vi "Select DaisyChain device.vi"(0 "System no.":i32=1 min=1 max=4 step=1, 1 "DLL Interface":T1=5 items=["RS232", "GPIB", "Board", "TCP-IP", "USB", "RS232_DC", "USB_DC", "TCPIP_DC"], 2 "Controller name":string, 3 "Timeout":i32=5000, 4 "Register DC":bool, 5 "error in":errorcluster, 6 "RS232 Portnumber":i32(ring) items=["COM1", "COM2", "COM3", "COM4", "COM5", "COM6", "COM7", "COM8", "COM9", "COM10", "COM11", "COM12", "COM13", "COM14", "COM15", "COM16", "COM17", "COM18", "COM19", "COM20", "COM21", "COM22", "COM23", "COM24", "COM25", "COM26", "COM27", "COM28", "COM29", "COM30"], 7 "RS232 Baud rate":i32=57600, 8 "Parameter":string) -> (14 "Selected DaisyChain controller":string, 15 "DeviceID out":i32, 19 "error out":errorcluster)   [LabVIEW 2026]
doc: "Performs a broadcast, returns names of all controllers matching Controller name and lets the user select the appropriate controller from a ring control. VI will also stop if Cancel is TRUE.\n\nC-867: Controller name = \"C-867\", DLL Interface = RS232_DC\nC-885: Controller name = \"C-885\", DLL Interface = USB_DC or TCPIP_DC\nE-709: Controller name = \"E-709\", DLL Interface = RS232_DC. Only supported if E-709 is used inside C-867K012/K013.\nE-755: Controller name = \"E-755\", DLL Interface = RS232_DC\nE-861: Controller name = \"E-861\", DLL Interface = RS232_DC or USB_DC\nE-871: Controller name = \"E-871\", DLL Interface = RS232_DC or USB_DC\nMercury_GCS: Controller name = \"Mercury_GCS\", DLL Interface = RS232_DC or USB_DC"
uses:
  Available DLL interfaces.ctl
  Available interfaces.ctl
  Available DLLs.ctl
  Global1.vi
  Global DaisyChain.vi
panel:
  in  "abort":bool
  in  "ok":bool
  in  "Please select DaisyChain controller":u16(ring) items=["DeviceID 1: (c)2013 Physik Instrumente (PI) GmbH & Co. KG, E-871.1A1, 0, 01.009 ", "DeviceID 2: <device 2 not connected> ", "DeviceID 3: <device 3 not connected> ", "DeviceID 4: <device 4 not connected> ", "DeviceID 5: <device 5 not connected> ", "DeviceID 6: <device 6 not connected> ", "DeviceID 7: <device 7 not connected> ", "DeviceID 8: <device 8 not connected> ", "DeviceID 9: (c)2013 Physik Instrumente (PI) GmbH & Co. KG, E-871.1A1, 0, 01.009 ", "DeviceID 10: <device 10 not connected> ", "DeviceID 11: <device 11 not connected> ", "DeviceID 12: <device 12 not connected> ", "DeviceID 13: <device 13 not connected> ", "DeviceID 14: <device 14 not connected> ", "DeviceID 15: <device 15 not connected> ", "DeviceID 16: <device 16 not connected> ", "DeviceID 17: <device 17 not connected>"]
  out "Please wait":string="Broadcast is running, please wait..."
  # "Scan parameters and controller name to search for:"
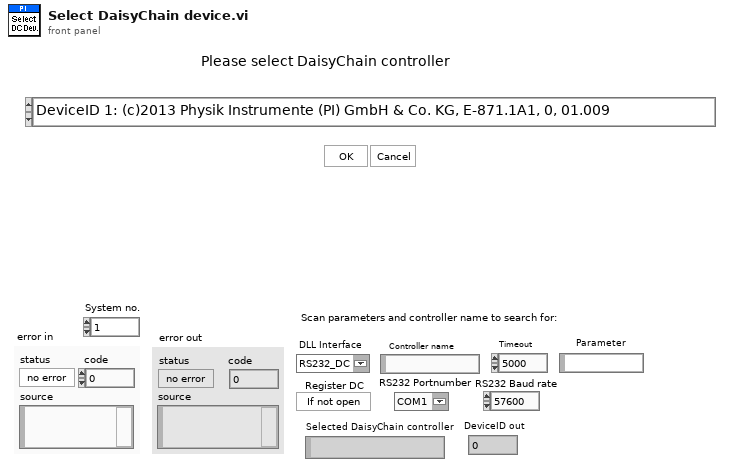
[diagram p1: front panel]
types:
  T1 = typedef "Available DLL interfaces.ctl" = u16
  T2 = enum16{"C844_IsDLLAvailable", "C844_ConnectRS232", "C844_ConnectNIgpib", "C844_IsConnected", "C844_CloseConnection", "C844_GcsCommandset", "C844_GetError", "C844_GcsGetAnswerSize", "C844_GcsGetAnswer", "C843_IsDLLAvailable", "C843_Connect", "C843_IsConnected", "C843_CloseConnection", "C843_GcsCommandset", "C843_GetError", "C843_GcsGetAnswerSize", "C843_GcsGetAnswer", "E710_IsDLLAvailable", "E710_ConnectRS232", "E710_ConnectNIgpib", "E710_IsConnected", "E710_CloseConnection", "E710_GcsCommandset", "E710_GetError", "E710_GcsGetAnswerSize", "E710_GcsGetAnswer", "C843_PM_IsDLLAvailable", "C843_PM_Connect", "C843_PM_IsConnected", "C843_PM_CloseConnection", "C843_PM_GcsCommandset", "C843_PM_GetError", "C843_PM_GcsGetAnswerSize", "C843_PM_GcsGetAnswer", "C843_PM_GetCurrentBoardID", "C843_GetCurrentBoardID", "C865_IsDLLAvailable", "C865_ConnectRS232", "C865_IsConnected", "C865_CloseConnection", "C865_GcsCommandset", "C865_GetError", "C865_GcsGetAnswerSize", "C865_GcsGetAnswer", "C865_GetCurrentInterfaceID", "E761_ConnectPciBoard", "DefineSystem", "CloseConnection", "IsConnected", "ConnectRS232", "ConnectNIgpib", "ConnectPciBoard", "ConnectTCPIP", "GetError", "GcsCommandset", "GCSGetAnswerSize", "GcsGetAnswer"}
  T3 = enum16{"C844_IsDLLAvailable", "C844_ConnectRS232", "C844_ConnectNIgpib", "C844_IsConnected", "C844_CloseConnection", "C844_GcsCommandset", "C844_GetError", "C844_GcsGetAnswerSize", "C844_GcsGetAnswer", "C843_IsDLLAvailable", "C843_Connect", "C843_IsConnected", "C843_CloseConnection", "C843_GcsCommandset", "C843_GetError", "C843_GcsGetAnswerSize", "C843_GcsGetAnswer", "E710_IsDLLAvailable", "E710_ConnectRS232", "E710_ConnectNIgpib", "E710_IsConnected", "E710_CloseConnection", "E710_GcsCommandset", "E710_GetError", "E710_GcsGetAnswerSize", "E710_GcsGetAnswer", "C843_PM_IsDLLAvailable", "C843_PM_Connect", "C843_PM_IsConnected", "C843_PM_CloseConnection", "C843_PM_GcsCommandset", "C843_PM_GetError", "C843_PM_GcsGetAnswerSize", "C843_PM_GcsGetAnswer", "C843_PM_GetCurrentBoardID", "C843_GetCurrentBoardID", "C865_IsDLLAvailable", "C865_ConnectRS232", "C865_IsConnected", "C865_CloseConnection", "C865_GcsCommandset", "C865_GetError", "C865_GcsGetAnswerSize", "C865_GcsGetAnswer", "C865_GetCurrentInterfaceID", "E761_ConnectPciBoard", "DefineSystem", "CloseConnection", "IsConnected", "ConnectRS232", "ConnectNIgpib", "ConnectPciBoard", "ConnectTCPIP", "GetError", "GcsCommandset", "GCSGetAnswerSize", "GcsGetAnswer", "CloseDaisyChain", "OpenRS232DaisyChain", "ConnectDaisyChainDevice", "ConnectUSB", "ListUSB", "OpenUSBDaisyChain", "OpenTCPIPDaisyChain"}
  T4 = typedef "Available interfaces.ctl" = u16
  T5 = typedef "Available DLLs.ctl" = u16
  T6 = cluster{"DLL for Device":T5, "DLL Interface":T1, "Parameter":string}[]
  T7 = cluster{"RS232 Portnumber":i32, "Timeout":i32, "RS232 Baud rate":u32, "Interface":T4, "GPIB Bus":i32, "GPIB Address":i32, "GPIB Mode":i32}[]
  T8 = cluster{"input XON/XOFF":bool, "input HW Handshake":bool, "input alt HW HShk":bool, "output XON/XOFF":bool, "output HW Handshake":bool, "output alt HW HShk":bool, "XOFF byte ":u8, "XON byte":u8, "parity error byte":u16}[]
  T9 = cluster{"RS232 Portnumber":i32, "Timeout":i32, "RS232 Baud rate":u32, "Interface":T4, "GPIB Bus":i32, "GPIB Address":i32, "GPIB Mode":i32}
  T10 = cluster{"DLL for Device":T5, "DLL Interface":T1, "Parameter":string}
  T11 = cluster{"input XON/XOFF":bool, "input HW Handshake":bool, "input alt HW HShk":bool, "output XON/XOFF":bool, "output HW Handshake":bool, "output alt HW HShk":bool, "XOFF byte ":u8, "XON byte":u8, "parity error byte":u16}
  T12 = cluster{"No. of devices":i32, "Port ID":i32, "Devices":string[], "Description":string}[]
  T13 = cluster{"No. of devices":i32, "Port ID":i32, "Devices":string[], "Description":string}
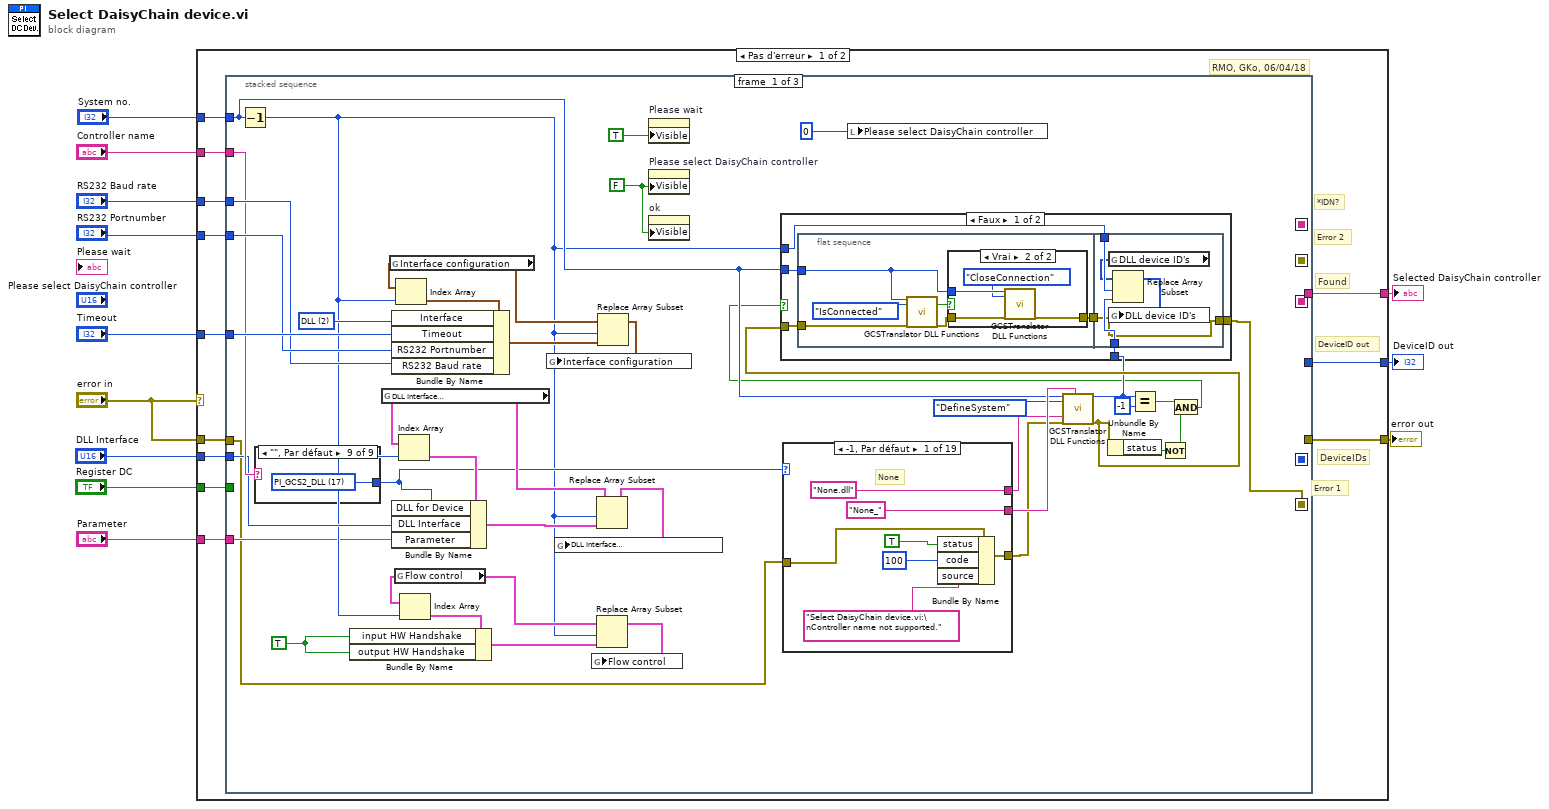
[diagram p0: block diagram]
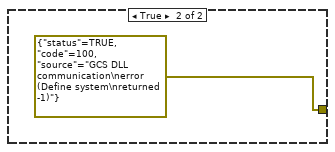
[diagram p3: hidden frame]
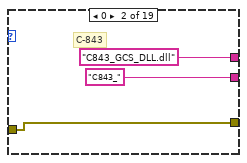
[diagram p4: hidden frame]
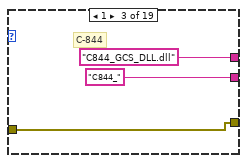
[diagram p5: hidden frame]
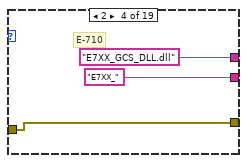
[diagram p6: hidden frame]
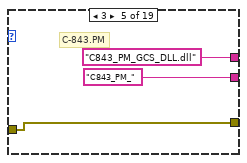
[diagram p7: hidden frame]
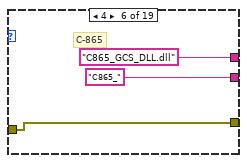
[diagram p8: hidden frame]
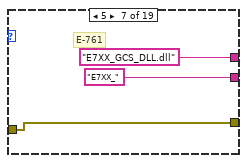
[diagram p9: hidden frame]
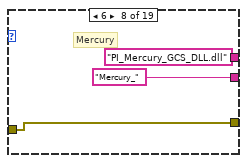
[diagram p10: hidden frame]
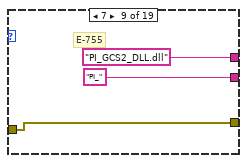
[diagram p11: hidden frame]
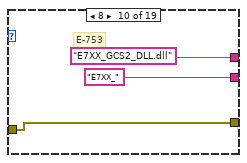
[diagram p12: hidden frame]
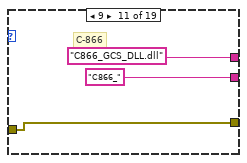
[diagram p13: hidden frame]
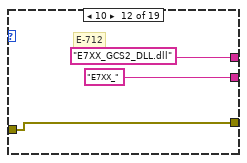
[diagram p14: hidden frame]
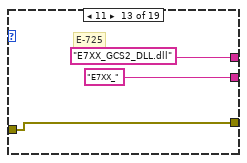
[diagram p15: hidden frame]
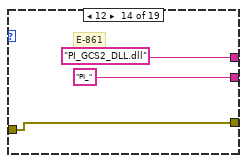
[diagram p16: hidden frame]
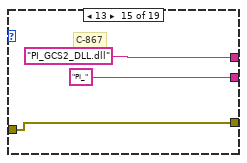
[diagram p17: hidden frame]
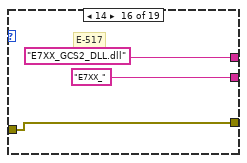
[diagram p18: hidden frame]
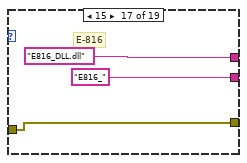
[diagram p19: hidden frame]
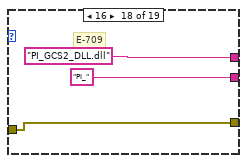
[diagram p20: hidden frame]
diagram:
  n1 = case shown="Pas d'erreur" "error in" {
    tunnel: [w21 w360] -> w12
    tunnel: "error in" -> [w22 w360]
    tunnel: "RS232 Baud rate" -> [w24 _]
    tunnel: "Controller name" -> [w23 _]
    tunnel: [w19 "" ("Host address/name")] -> w8
    tunnel: "RS232 Portnumber" -> [w20 _]
    tunnel: [w18 0] -> w7
    tunnel: "Register DC" -> [w17 _]
    tunnel: "System no." -> [w16 _]
    tunnel: "Timeout" -> [w15 _]
    tunnel: "DLL Interface" -> [w14 _]
    tunnel: "Parameter" -> [w13 _]
    frame No Error {
      # "DeviceIDs"
      # "Error 1"
      # "DeviceID out"
      # "Error 2"
      # "Found"
      # "*IDN?"
      # "RMO, GKo, 06/04/18"
      n2 = stacked-sequence {
        seq-local: [_ w163 _] -> [_ _ w304]
        seq-local: [_ w165 _] -> [_ _ w307]
        seq-local: [_ w161 _] -> [_ _ w302]
        seq-local: [w29 _ _] -> [_ w157 _]
        seq-local: [_ w159 _] -> [_ _ w301]
        tunnel: w24 -> [w53 _ _]
        tunnel: w23 -> [w51 w164 _]
        tunnel: w22 -> [w26 _ _]
        tunnel: [_ _ w303] -> w21
        tunnel: [_ _ w306] -> w19
        tunnel: w20 -> [w54 _ _]
        tunnel: [_ _ w305] -> w18
        tunnel: w17 -> [_ w162 _]
        tunnel: w16 -> [w33 w160 _]
        tunnel: w15 -> [w58 _ _]
        tunnel: w14 -> [w50 w158 _]
        tunnel: w13 -> [w27 _ _]
        frame #0 {
          w43 = FALSE ("Visible")
          w62 = T4 2 items=["RS232", "GPIB", "DLL", "TCP-IP"] ("Interface")
          w60 = TRUE ("Bundle Element")
          n3 = Decrement(x=w33) -> (x-1=w31:i32)
          n4 = case shown="\"\", Par défaut" w51 {
            tunnel: [-1 w149 w150 w151 w152 w153 w154 w155 w156] -> w37
            frame "None" {
            }
            frame "E-755" {
              w149 = T5 7 items=["C-843", "C-844", "E-710", "C-843.PM", "C-865", "E-761", "Mercury", "E-755", "E-753", "C-866", "E-712", "E-725", "E-861", "C-867", "E-517", "E-816", "E-709", "PI_GCS2_DLL", "HydraPollux"] ("DLL for Device")
            }
            frame "E-861" {
              w150 = T5 12 items=["C-843", "C-844", "E-710", "C-843.PM", "C-865", "E-761", "Mercury", "E-755", "E-753", "C-866", "E-712", "E-725", "E-861", "C-867", "E-517", "E-816", "E-709", "PI_GCS2_DLL", "HydraPollux"] ("DLL for Device")
            }
            frame "E-709" {
              w151 = T5 17 items=["C-843", "C-844", "E-710", "C-843.PM", "C-865", "E-761", "Mercury", "E-755", "E-753", "C-866", "E-712", "E-725", "E-861", "C-867", "E-517", "E-816", "E-709", "PI_GCS2_DLL", "HydraPollux"] ("DLL for Device")
            }
            frame "C-867" {
              w152 = T5 13 items=["C-843", "C-844", "E-710", "C-843.PM", "C-865", "E-761", "Mercury", "E-755", "E-753", "C-866", "E-712", "E-725", "E-861", "C-867", "E-517", "E-816", "E-709", "PI_GCS2_DLL", "HydraPollux"] ("DLL for Device")
            }
            frame "Mercury_GCS" {
              w153 = T5 17 items=["C-843", "C-844", "E-710", "C-843.PM", "C-865", "E-761", "Mercury", "E-755", "E-753", "C-866", "E-712", "E-725", "E-861", "C-867", "E-517", "E-816", "E-709", "PI_GCS2_DLL", "HydraPollux"] ("DLL for Device")
            }
            frame "E-871" {
              w154 = T5 17 items=["C-843", "C-844", "E-710", "C-843.PM", "C-865", "E-761", "Mercury", "E-755", "E-753", "C-866", "E-712", "E-725", "E-861", "C-867", "E-517", "E-816", "E-709", "PI_GCS2_DLL", "HydraPollux"] ("DLL for Device")
            }
            frame "C-885" {
              w155 = T5 17 items=["C-843", "C-844", "E-710", "C-843.PM", "C-865", "E-761", "Mercury", "E-755", "E-753", "C-866", "E-712", "E-725", "E-861", "C-867", "E-517", "E-816", "E-709", "PI_GCS2_DLL", "HydraPollux"] ("DLL for Device")
            }
            frame "", Default {
              w156 = T5 17 items=["C-843", "C-844", "E-710", "C-843.PM", "C-865", "E-761", "Mercury", "E-755", "E-753", "C-866", "E-712", "E-725", "E-861", "C-867", "E-517", "E-816", "E-709", "PI_GCS2_DLL", "HydraPollux"] ("DLL for Device")
            }
          }
          n5 = global read "Global1.vi" "DLL Interface\nConfiguration"() -> (w46:T6)
          n6 = global read "Global1.vi" "Interface configuration"() -> (w47:T7)
          n7 = global read "Global1.vi" "Flow control"() -> (w45:T8)
          n8 = Index Array(array=w47, index=w31) -> (element=w63:T9)
          n9 = Bundle By Name(cluster=w63, "Interface"=w62, "Timeout"=w58, "RS232 Portnumber"=w54, "RS232 Baud rate"=w53) -> (w52:T9)
          n10 = Index Array(array=w46, index=w31) -> (element=w59:T10)
          n11 = Bundle By Name(cluster=w59, "DLL for Device"=w37, "DLL Interface"=w50, "Parameter"=w27) -> (w49:T10)
          n12 = Index Array(array=w45, index=w31) -> (element=w61:T11)
          n13 = Bundle By Name(cluster=w61, "input HW Handshake"=w60, "output HW Handshake"=w60) -> (w48:T11)
          n14 = Replace Array Subset(array=w46, new element=w49, index=w31) -> (w56:T6)
          n15 = global write "Global1.vi" "DLL Interface\nConfiguration"(w56) -> ()
          n16 = Replace Array Subset(array=w45, new element=w48, index=w31) -> (w57:T8)
          n17 = global write "Global1.vi" "Flow control"(w57) -> ()
          n18 = Replace Array Subset(array=w47, new element=w52, index=w31) -> (w55:T7)
          n19 = global write "Global1.vi" "Interface configuration"(w55) -> ()
          n20 = property on="Please wait" class="Ch"("Visible"=TRUE) -> ()  [unwired: 2 in, 2 out]
          n21 = property on="Please select DaisyChain controller" class="MDér (strict)"("Visible"=w43) -> ()  [unwired: 2 in, 2 out]
          n22 = property on="ok" class="Bool"("Visible"=w43) -> ()  [unwired: 2 in, 2 out]
          n23 = case shown="-1, Par défaut" w37 {
            tunnel: ["None.dll" "C843_GCS_DLL.dll" "C844_GCS_DLL.dll" "E7XX_GCS_DLL.dll" "C843_PM_GCS_DLL.dll" "C865_GCS_DLL.dll" "E7XX_GCS_DLL.dll" "PI_Mercury_GCS_DLL.dll" "PI_GCS2_DLL.dll" "E7XX_GCS2_DLL.dll" "C866_GCS_DLL.dll" "E7XX_GCS2_DLL.dll" "E7XX_GCS2_DLL.dll" "PI_GCS2_DLL.dll" "PI_GCS2_DLL.dll" "E7XX_GCS2_DLL.dll" "E816_DLL.dll" "PI_GCS2_DLL.dll" "PI_GCS2_DLL.dll"] -> w40
            tunnel: ["None_" "C843_" "C844_" "E7XX_" "C843_PM_" "C865_" "E7XX_" "Mercury_" "PI_" "E7XX_" "C866_" "E7XX_" "E7XX_" "PI_" "PI_" "E7XX_" "E816_" "PI_" "PI_"] -> w41
            tunnel: w26 -> [w87 w94 w97 w100 w103 w106 w109 w112 w115 w118 w121 w124 w127 w130 w133 w136 w139 w142 w145]
            tunnel: [w91 w94 w97 w100 w103 w106 w109 w112 w115 w118 w121 w124 w127 w130 w133 w136 w139 w142 w145] -> w25
            frame -1, Default {
              # "None"
              n24 = Bundle By Name(cluster=w87, "status"=TRUE, "code"=100, "source"="Select DaisyChain device.vi:\nController name not supported.") -> (w91:errorcluster)
            }
            frame 0 {
              # "C-843"
            }
            frame 1 {
              # "C-844"
            }
            frame 2 {
              # "E-710"
            }
            frame 3 {
              # "C-843.PM"
            }
            frame 4 {
              # "C-865"
            }
            frame 5 {
              # "E-761"
            }
            frame 6 {
              # "Mercury"
            }
            frame 7 {
              # "E-755"
            }
            frame 8 {
              # "E-753"
            }
            frame 9 {
              # "C-866"
            }
            frame 10 {
              # "E-712"
            }
            frame 11 {
              # "E-725"
            }
            frame 12 {
              # "E-861"
            }
            frame 13 {
              # "C-867"
            }
            frame 14 {
              # "E-517"
            }
            frame 15 {
              # "E-816"
            }
            frame 16 {
              # "E-709"
            }
            frame 17 {
              # "PI_GCS2_DLL"
            }
          }
          n25 = local write "Please select DaisyChain controller"(0) -> ()
          n26 = call "GCSTranslator DLL Functions.vi"("System no."=w33, "Function"=T2."DefineSystem", "String input"=w40, "error in"=w25, "String input 2"=w41) -> ("DLL I32 Return value"=w30:i32, "error out"=w32:errorcluster)  [unwired: 2 in, 11 out]
          n27 = Unbundle By Name(w32) -> ("status"=w35:bool)
          n28 = Equal?(x=w30, y=-1) -> (x = y?=w36:bool)
          n29 = Not(x=w35) -> (.not. x?=w34:bool)
          n30 = And(x=w36, y=w34) -> (x .and. y?=w28:bool)
          n31 = case shown="Faux" w28 {
            tunnel: w33 -> [w64 _]
            tunnel: w32 -> [w67 _]
            tunnel: w31 -> [w69 _]
            tunnel: w30 -> [w68 _]
            tunnel: [w65 errorcluster {"status"=TRUE, "code"=100, "source"="GCS DLL communication\nerror (Define system\nreturned -1)"} ("error out")] -> w29
            frame False {
              n32 = flat-sequence {
                tunnel: w67 -> [w72]
                tunnel: [w71] -> w66
                tunnel: w64 -> [w70]
                tunnel: w69 -> [w85]
                tunnel: w68 -> [w82]
                tunnel: w66 -> [w81]
                tunnel: [w81] -> w65
                frame #0 {
                  n33 = call "GCSTranslator DLL Functions.vi"("System no."=w70, "Function"=T2."IsConnected", "error in"=w72) -> ("Boolean output"=w75:bool, "error out"=w74:errorcluster)  [unwired: 4 in, 11 out]
                  n34 = case shown="Vrai" w75 {
                    tunnel: w70 -> [_ w80]
                    tunnel: w74 -> [w76 w79]
                    tunnel: [w76 w78] -> w71
                    frame False {
                    }
                    frame True {
                      n35 = call "GCSTranslator DLL Functions.vi"("System no."=w80, "Function"=T2."CloseConnection", "error in"=w79) -> ("error out"=w78:errorcluster)  [unwired: 4 in, 12 out]
                    }
                  }
                }
                frame #1 {
                  n36 = global read "Global1.vi" "DLL device ID's"() -> (w83:i32[])
                  n37 = Replace Array Subset(array=w83, new element=w82, index=w85) -> (w84:i32[])
                  n38 = global write "Global1.vi" "DLL device ID's"(w84) -> ()
                }
              }
            }
            frame True {
            }
          }
        }
        frame #1 {
          n39 = case shown="Pas d'erreur" w157 {
            tunnel: [w181 string[] []] -> w165
            tunnel: w164 -> [w167 _]
            tunnel: [w180 w300] -> w163
            tunnel: w162 -> [w179 _]
            tunnel: [w178 string[] []] -> w161
            tunnel: w160 -> [w173 _]
            tunnel: [w172 i32[] []] -> w159
            tunnel: w158 -> [w171 _]
            tunnel: w157 -> [w168 w300]
            frame No Error {
              n40 = Decrement(x=w173) -> (x-1=w177:i32)
              n41 = case shown="Vrai" w179 {
                tunnel: w168 -> [w256 w288]
                tunnel: [w252 w281] -> w170
                tunnel: w173 -> [w254 w286]
                tunnel: [w251 w283] -> w175
                tunnel: w177 -> [w250 _]
                tunnel: [w249 w284] -> w176
                tunnel: w171 -> [w248 w282]
                frame False {
                  n42 = call "Is DaisyChain open.vi"("System no."=w254, "error in"=w256) -> ("DC open?"=w255:bool, "error out"=w253:errorcluster)  [unwired: 16 out]
                  n43 = case shown="Faux" w255 {
                    tunnel: w254 -> [_ w270]
                    tunnel: w253 -> [w262 w269]
                    tunnel: [w262 w268] -> w252
                    tunnel: [w259 w267] -> w251
                    tunnel: w250 -> [w258 _]
                    tunnel: [w257 w265] -> w249
                    tunnel: w248 -> [_ w263]
                    frame True {
                      n44 = global read "Global DaisyChain.vi" "DaisyChain configuration"() -> (w260:T12)
                      n45 = Index Array(array=w260, index=w258) -> (element=w261:T13)
                      n46 = Unbundle By Name(w261) -> ("Port ID"=w259:i32, "Devices"=w257:string[])
                    }
                    frame False {
                      n47 = case shown="7" w263 {
                        tunnel: [T3."OpenRS232DaisyChain" ("Function") T3."OpenRS232DaisyChain" ("Function") T3."OpenRS232DaisyChain" ("Function") T3."OpenRS232DaisyChain" ("Function") T3."OpenRS232DaisyChain" ("Function") T3."OpenRS232DaisyChain" ("Function") T3."OpenUSBDaisyChain" ("Function") T3."OpenTCPIPDaisyChain" ("Function")] -> w264
                        frame 0, Default {
                        }
                        frame 1 {
                        }
                        frame 2 {
                        }
                        frame 3 {
                        }
                        frame 4 {
                        }
                        frame 5 {
                        }
                        frame 6 {
                        }
                        frame 7 {
                        }
                      }
                      n48 = call "GCSTranslator DLL Functions.vi"("System no."=w270, "Function"=w264, "error in"=w269) -> ("DLL I32 Return value"=w267:i32, "String output"=w266:string, "error out"=w268:errorcluster)  [unwired: 4 in, 10 out]
                      n49 = call "Get lines from string.vi"("Input string"=w266) -> ("Strings"=w265:string[])  [unwired: 2 in, 16 out]
                    }
                  }
                }
                frame True {
                  n50 = case shown="7" w282 {
                    tunnel: [T3."OpenRS232DaisyChain" ("Function") T3."OpenRS232DaisyChain" ("Function") T3."OpenRS232DaisyChain" ("Function") T3."OpenRS232DaisyChain" ("Function") T3."OpenRS232DaisyChain" ("Function") T3."OpenRS232DaisyChain" ("Function") T3."OpenUSBDaisyChain" ("Function") T3."OpenTCPIPDaisyChain" ("Function")] -> w280
                    frame 0, Default {
                    }
                    frame 1 {
                    }
                    frame 2 {
                    }
                    frame 3 {
                    }
                    frame 4 {
                    }
                    frame 5 {
                    }
                    frame 6 {
                    }
                    frame 7 {
                    }
                  }
                  n51 = call "GCSTranslator DLL Functions.vi"("System no."=w286, "Function"=T3."CloseDaisyChain", "error in"=w288) -> ("error out"=w287:errorcluster)  [unwired: 4 in, 12 out]
                  n52 = call "GCSTranslator DLL Functions.vi"("System no."=w286, "Function"=w280, "error in"=w287) -> ("DLL I32 Return value"=w283:i32, "String output"=w285:string, "error out"=w281:errorcluster)  [unwired: 4 in, 10 out]
                  n53 = call "Get lines from string.vi"("Input string"=w285) -> ("Strings"=w284:string[])  [unwired: 2 in, 16 out]
                }
              }
              n54 = case shown="\"Mercury_GCS\"" w167 {
                tunnel: [w183 string[] ["C-663", "C-863"]] -> w166
                tunnel: w167 -> [w182 _]
                frame Default {
                  n55 = Build Array(w182) -> (w183:string[])
                }
                frame "Mercury_GCS" {
                }
              }
              n56 = Not Equal?(x=w175, y=-1) -> (x != y?=w169:bool)
              n57 = case shown="Vrai" w169 {
                tunnel: [string[] [] w207] -> w181
                tunnel: w166 -> [_ w202]
                tunnel: [w187 w201] -> w180
                tunnel: [string[] [] w200] -> w178
                tunnel: w170 -> [w192 w199]
                tunnel: w176 -> [_ w198]
                tunnel: w173 -> [w191 _]
                tunnel: [i32[] [] w193] -> w172
                frame False {
                  # "Error!"
                  n58 = call "GCSTranslator DLL Functions.vi"("System no."=w191, "Function"=T3."GetError", "error in"=w192) -> ("error out"=w188:errorcluster)  [unwired: 4 in, 12 out]
                  n59 = call "GCSTranslateError.vi"("error in"=w188) -> ("error out"=w187:errorcluster)  [unwired: 18 out]
                }
                frame True {
                  n60 = for {
                    tunnel: w202 -> [w214] mode=indexing
                    tunnel: w198 -> [w212]
                    shift-right: [w213] -> w200
                    shift-left: string[] [] -> [w215]
                    shift-right: [w210] -> w194
                    shift-left: i32[] [] -> [w211]
                    n61 = for {
                      tunnel: w212 -> [w223] mode=indexing
                      shift-right: [w222] -> w213
                      shift-left: w215 -> [w221]
                      tunnel: w214 -> [w220]
                      shift-right: [w219] -> w210
                      shift-left: w211 -> [w218]
                      i -> [w216]
                      n62 = Match Pattern(string=w223, regular expression=w220) -> (offset past match=w217:i32)  [unwired: 4 out]
                      n63 = Not Equal?(x=w217, y=-1) -> (x != y?=w224:bool)
                      n64 = case shown="Vrai" w224 {
                        tunnel: w223 -> [_ w232]
                        tunnel: [w227 w233] -> w222
                        tunnel: w221 -> [w227 w231]
                        tunnel: [w226 w230] -> w219
                        tunnel: w218 -> [w226 w229]
                        tunnel: w216 -> [_ w228]
                        frame False {
                        }
                        frame True {
                          n65 = Build Array (concatenate)(w229, w228) -> (w230:i32[])
                          n66 = Build Array (concatenate)(w231, w232) -> (w233:string[])
                        }
                      }
                    }
                  }
                  n67 = Array Size(array=w200) -> (size(s)=w206:i32)
                  n68 = Array Size(array=w200) -> (size(s)=w204:i32)
                  n69 = Increment(x=w194) -> (x+1=w193:i32[])
                  n70 = Equal To 0?(x=w204) -> (x = 0?=w203:bool)
                  n71 = Initialize Array("", w206) -> (w209:string[])
                  n72 = case shown="Faux" w203 {
                    tunnel: [w234 w236] -> w201
                    tunnel: w199 -> [w234 w235]
                    frame False {
                    }
                    frame True {
                      n73 = Bundle By Name(cluster=w235, "status"=TRUE, "code"=100 ("Bundle Element"), "source"="Controller not found" ("Bundle Element")) -> (w236:errorcluster)
                    }
                  }
                  n74 = Number To Decimal String(number=w193, width (-)=i16 0) -> (decimal integer string=w195:string[])
                  n75 = for {
                    N: w206 -> [_]
                    shift-right: [w245] -> w207
                    shift-left: w209 -> [w247]
                    tunnel: w200 -> [w241] mode=indexing
                    tunnel: w195 -> [w240] mode=indexing
                    i -> [w243]
                    n76 = Concatenate Strings("DeviceID ", w240, ": " ("string"), w241) -> (w246:string)
                    n77 = Replace Array Subset(array=w247, new element=w246, index=w243) -> (w245:string[])
                  }
                }
              }
            }
            frame Error {
            }
          }
        }
        frame #2 {
          n78 = case shown="Pas d'erreur" w304 {
            tunnel: w307 -> [w319 _]
            tunnel: w302 -> [w318 _]
            tunnel: [w317 "" ("Host address/name")] -> w306
            tunnel: [w315 0] -> w305
            tunnel: w304 -> [w313 w354]
            tunnel: [w309 w354] -> w303
            tunnel: w301 -> [w308 _]
            frame No Error {
              n79 = flat-sequence {
                tunnel: w319 -> [w321]
                tunnel: w313 -> [w320]
                tunnel: [w320] -> w312
                tunnel: w312 -> [w323]
                tunnel: [w323] -> w311
                tunnel: w318 -> [w330]
                tunnel: [w329] -> w316
                tunnel: [w328] -> w314
                tunnel: w311 -> [w327]
                tunnel: [w326] -> w310
                tunnel: w308 -> [w325]
                tunnel: [w353] -> w317
                tunnel: w316 -> [w353]
                tunnel: [w351] -> w315
                tunnel: w314 -> [w351]
                tunnel: [w350] -> w309
                tunnel: w310 -> [w350]
                frame #0 {
                  n80 = property on="Please select DaisyChain controller" class="MDér (strict)"("Strings []"=w321) -> ()  [unwired: 2 in, 2 out]
                  n81 = property on="Please wait" class="Ch"("Visible"=FALSE) -> ()  [unwired: 2 in, 2 out]
                }
                frame #1 {
                  w324 = TRUE ("Visible")
                  n82 = property on="Please select DaisyChain controller" class="MDér (strict)"("Visible"=w324) -> ()  [unwired: 2 in, 2 out]
                  n83 = property on="ok" class="Bool"("Visible"=w324) -> ()  [unwired: 2 in, 2 out]
                }
                frame #2 {
                  n84 = while {
                    tunnel: w330 -> [w338]
                    tunnel: [w337] -> w329
                    tunnel: [w336] -> w328
                    tunnel: w327 -> [w335]
                    tunnel: [w334] -> w326
                    tunnel: w325 -> [w331]
                    stop <- w340 stop-if-true
                    n85 = case shown="Faux" "abort" {
                      tunnel: w335 -> [w341 _]
                      tunnel: [w341 errorcluster {"status"=TRUE, "code"=100, "source"="Select DaisyChain device was canceled"} ("error out")] -> w334
                      frame False {
                      }
                      frame True {
                      }
                    }
                    n86 = case shown="Vrai" "ok" {
                      tunnel: w338 -> [_ w349]
                      tunnel: ["" ("Host address/name") w348] -> w337
                      tunnel: [0 w345] -> w336
                      tunnel: w331 -> [_ w346]
                      frame False {
                      }
                      frame True {
                        n87 = local read "Please select DaisyChain controller"() -> (w347:u16)
                        n88 = Index Array(array=w349, index=w347) -> (element=w348:string)
                        n89 = Index Array(array=w346, index=w347) -> (element=w345:i32)
                      }
                    }
                    n90 = Or(x="ok", y="abort") -> (x .or. y?=w340:bool)
                    n91 = Wait Until Next ms Multiple(millisecond multiple=u32 10) -> ()  [unwired: 1 out]
                  }
                }
                frame #3 {
                  n92 = local write "abort"(FALSE ("abort")) -> ()
                }
              }
            }
            frame Error {
              n93 = One Button Dialog(message="Error! \nController not found.\nPlease check settings and retry.") -> ()  [unwired: 2 out]
            }
          }
        }
      }
    }
    frame Error {
    }
  }
  "error out" <- w12
  "Selected DaisyChain controller" <- w8
  "DeviceID out" <- w7
